vi "ConfigureSweepCoupling.vi"(8 "error in (no error)":errorcluster, 11 "Keysight44xx in":refnum<class "Keysight44xx.lvclass">) -> (0 "error out":errorcluster, 3 "Keysight44xx out":refnum<class "Keysight44xx.lvclass">)   [LabVIEW 2018, in "SpecAnPlugins.lvlib" / "Keysight44xx.lvclass"]
doc: "This function configures the coupling and sweeping attributes such as sweep time (time it takes to go from the start frequency to the stop frequency), Resolution Bandwidthm, and the Video Bandwidth."
uses:
  Keysight44xx.lvclass
  C:/Users/ico/Documents/Projects/NistPluggableModules/SpecAn/SpecAnPlugins/SpecAnBaseClass/SpecAnBase.lvclass
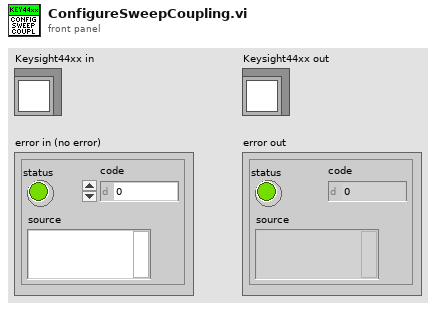
[diagram p1: front panel]
types:
  T1 = typedef "SpecAnPlugins.lvlib/SpecAnBase.lvclass/Acquisition.ctl" = cluster{"Handle":string, "Connected":bool, "Enabled":bool, "SweepModeContinuous":bool, "NumberOfSweeps":i32, "DetectorTypeAuto":bool, "DetectorType":i32, "VerticalScale":i32, "MaximumTime(seconds)":dbl}
  T2 = typedef "SpecAnPlugins.lvlib/SpecAnBase.lvclass/SweepCoupling.ctl" = cluster{"ResolutionBandwidth":dbl, "ResolutionBandwidthAuto":bool, "SweepTime":dbl, "VideoBandwidth":dbl, "VideoBandwidthAuto":bool, "SweepTimeAuto":bool}
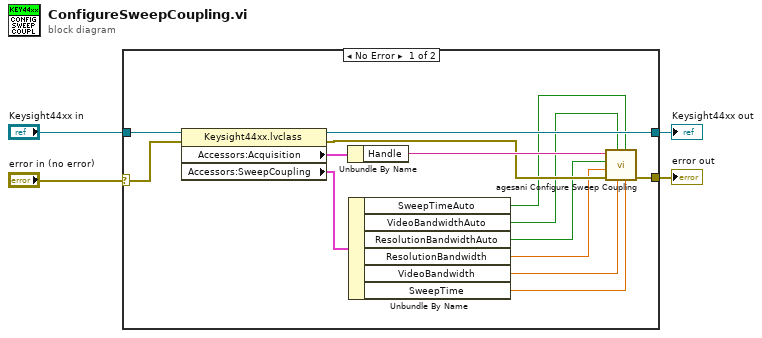
[diagram p0: block diagram]
diagram:
  n1 = case shown="No Error" "error in (no error)" {
    selector: "error in (no error)" -> [w17 w20]
    tunnel: [w11 w20] -> w3
    tunnel: "Keysight44xx in" -> [w18 w19]
    tunnel: [w16 w19] -> w1
    frame No Error {
      n2 = property class="Keysight44xx.lvclass"(reference=w18, error in=w17) -> (reference out=w16:refnum<class "Keysight44xx.lvclass">, error out=w12:errorcluster, "Accessors:Acquisition"=w15:T1, "Accessors:SweepCoupling"=w14:T2)
      n3 = Unbundle By Name(w15) -> ("Handle"=w13:string)
      n4 = Unbundle By Name(w14) -> ("SweepTimeAuto"=w5:bool, "VideoBandwidthAuto"=w6:bool, "ResolutionBandwidthAuto"=w7:bool, "ResolutionBandwidth"=w8:dbl, "VideoBandwidth"=w9:dbl, "SweepTime"=w10:dbl)
      n5 = call <instrlib>:"agesani Configure Sweep Coupling.vi"("sweep time (4.0e-3)"=w10, "sweep time auto (On)"=w5, "video bandwidth (3.0e6)"=w9, "video bandwidth auto (On)"=w6, "error in (no error)"=w12, "resolution bandwidth (3.0e6)"=w8, "resolution bandwidth auto (On)"=w7, "instrument handle"=w13) -> ("error out"=w11:errorcluster)  [unwired: 3 out]
    }
    frame Error {
    }
  }
  "error out" <- w3
  "Keysight44xx out" <- w1
